vi "Read permission.vi"(8 "error in (no error)":errorcluster, 11 "Person in":refnum<class "Person.lvclass">) -> (0 "error out":errorcluster, 2 "permission":T1=enum."User", 3 "Person out":refnum<class "Person.lvclass">)   [LabVIEW 2014, in "Person.lvclass"]
uses:
  Person.lvclass
  DEF-Permission.ctl
  Person.lvclass/Person.ctl
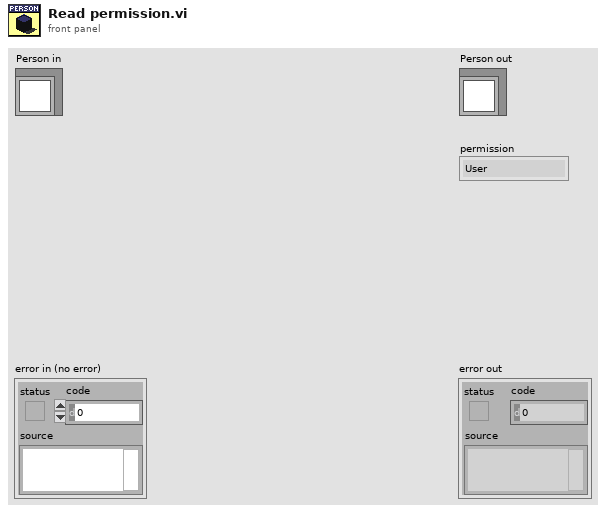
[diagram p1: front panel]
types:
  T1 = typedef "Person.lvclass/DEF-Permission.ctl" = enum16{"Visitor", "User", "Admin"}
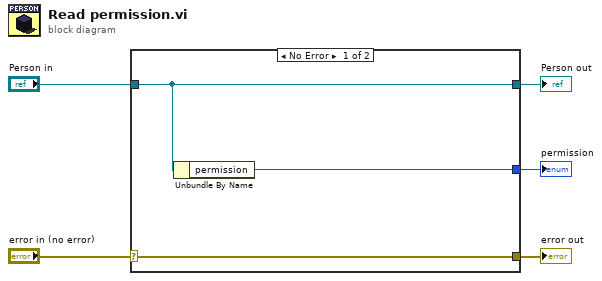
[diagram p0: block diagram]
diagram:
  n1 = case shown="No Error" "error in (no error)" {
    selector: "error in (no error)" -> [w8 w9]
    tunnel: [w8 w9] -> w4
    tunnel: [w7 w10] -> w2
    tunnel: "Person in" -> [w7 w10]
    tunnel: [w6 _] -> w1
    frame No Error {
      n2 = Unbundle By Name(w7) -> ("permission"=w6:T1)
    }
    frame Error {
    }
  }
  "error out" <- w4
  "Person out" <- w2
  "permission" <- w1
